vi "FPGA_ADC_read.vi"(2 "Readout parameter":T2, 3 "FPGA In":T1) -> (0 "data out":dbl[][](array[numeric]), 1 "FPGA Out":T1)   [LabVIEW 2013]
uses:
  fpga-bitfile-ref.ctl
  <vilib>/rvi/interface/common/niFpgaWaitOnOcc.vi
  <vilib>/Utility/error.llb/Error Cluster From Error Code.vi
  <vilib>/rvi/errors/niLvFpgaAdjustHostInterfaceError.vi
  <vilib>/rvi/interface/nirviMethod/nirviMethod.xnode
  FPGA Bitfiles/fpgabatch18_sbRIO9612RIO0_FPGAMAINlock-in_BbNldMosBaM.lvbitx
  <vilib>/FPGAPlugInAG/sbRIO-9612/niLvFpga_ReadFifo_sbRIO-9612.vi
  <vilib>/rvi/errors/niLvFpgaMergeErrorWithErrorCode.vi
panel:
  in  "stop read":bool
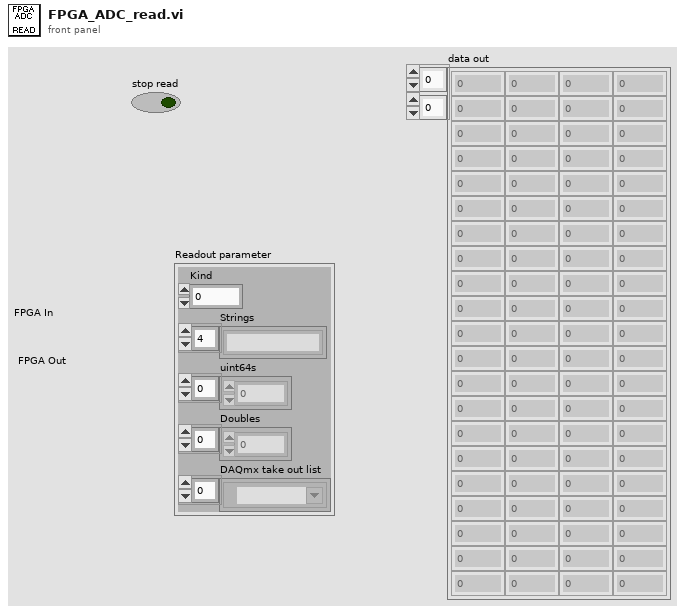
[diagram p1: front panel]
types:
  T1 = typedef "fpga-bitfile-ref.ctl" = refnum<k20>
  T2 = cluster{"Kind":u16, "Strings":string[], "uint64s":u64[], "Doubles":dbl[], "DAQmx take out list":refnum<k21>[]}
  T3 = enum16{"empty", "stop", "start", "sampling rate", "trigger", "sample count", "reset channels", "add channel", "avg per point", "manual trigger"}
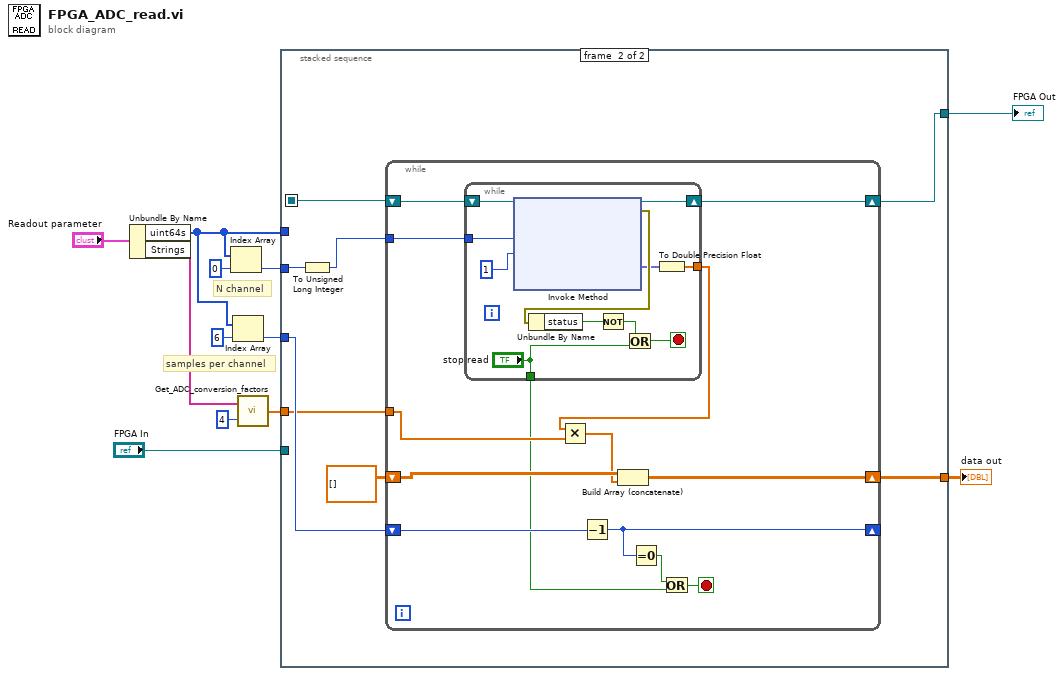
[diagram p0: block diagram]
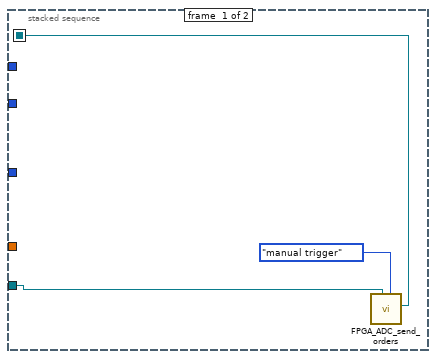
[diagram p2: hidden frame]
diagram:
  # "samples per channel"
  # "N channel"
  n1 = Unbundle By Name("Readout parameter") -> ("uint64s"=w7:u64[], "Strings"=w4:string[])
  n2 = Index Array(array=w7, index=0) -> (element=w10:u64)
  n3 = Index Array(array=w7, index=6) -> (element=w6:u64)
  n4 = call "Get_ADC_conversion_factors.vi"("index"=4, "Strings"=w4) -> ("elements"=w3:dbl[])
  n5 = stacked-sequence {
    seq-local: [w14 _] -> [_ w18]
    tunnel: w7 -> [_ _]
    tunnel: "FPGA In" -> [w13 _]
    tunnel: w10 -> [_ w23]
    tunnel: w6 -> [_ w21]
    tunnel: w3 -> [_ w20]
    tunnel: [_ w17] -> w2
    tunnel: [_ w16] -> w1
    frame #0 {
      n6 = call "FPGA_ADC_send_orders.vi"("option"=T3."manual trigger", "FPGA VI Reference In"=w13) -> ("FPGA VI Reference Out"=w14:T1)  [unwired: 8 in, 1 out]
    }
    frame #1 {
      n7 = To Unsigned Long Integer(number=w23) -> (unsigned 32bit integer=w22:u32)
      n8 = while {
        shift-right: [w33] -> w17
        shift-left: dbl[][] [] -> [w36]
        shift-right: [w34] -> w16
        shift-left: w18 -> [w35]
        tunnel: w22 -> [w32]
        shift-right: [w24] -> _
        shift-left: w21 -> [w28]
        tunnel: w20 -> [w30]
        stop <- w25 stop-if-true
        n9 = while {
          tunnel: [w40] -> w31
          shift-right: [w46] -> w34
          shift-left: w35 -> [w41]
          tunnel: w32 -> [w38]
          tunnel: ["stop read"] -> w27
          stop <- w42 stop-if-true
          n10 = xnode "Invoke Method"("FPGA VI Reference In"=w41, "Number of Elements"=w38, "Timeout (ms)"=1) -> ("FPGA VI Reference Out"=w46:T1, "error out"=w45:errorcluster, "Data"=w39:fxp<+/-,26,5>[])  [unwired: 1 in, 1 out]
          n11 = Unbundle By Name(w45) -> ("status"=w44:bool)
          n12 = Not(x=w44) -> (.not. x?=w43:bool)
          n13 = Or(x=w43, y="stop read") -> (x .or. y?=w42:bool)
          n14 = To Double Precision Float(number=w39) -> (double precision float=w40:dbl[])
        }
        n15 = Multiply(x=w31, y=w30) -> (x*y=w29:dbl[])
        n16 = Decrement(x=w28) -> (x-1=w24:u64)
        n17 = Build Array (concatenate)(w36, w29) -> (w33:dbl[][])
        n18 = Equal To 0?(x=w24) -> (x = 0?=w26:bool)
        n19 = Or(x=w26, y=w27) -> (x .or. y?=w25:bool)
      }
    }
  }
  "FPGA Out" <- w1
  "data out" <- w2
